vi "DriveModuleOpen.vi"(6 "Magnet Offset (Degrees)":dbl, 7 "ModualNamePrefix":string, 8 "error in":errorcluster, 9 "EncoderCanID":u8, 10 "SpinCanID":u8, 11 "TravelCanID":u8) -> (0 "error out":errorcluster)   [LabVIEW 2023]
uses:
  <vilib>/Rock Robotics/WPI/ThirdParty/REV Robotics/REVLib/Typedef/Spark MAX Idle Mode.ctl
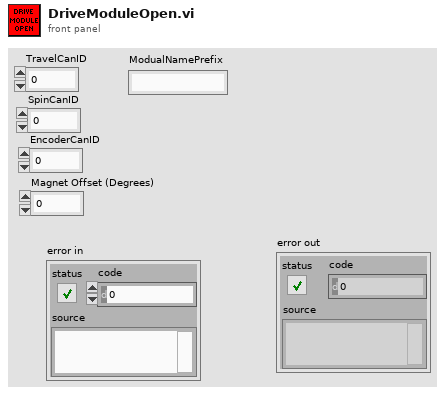
[diagram p1: front panel]
types:
  T1 = typedef "Spark MAX Idle Mode.ctl" = enum16{"Coast", "Brake"}
  T2 = typedef "CTRE_Phoenix_CANcoder_DeviceRef.ctl" = cluster{"DeviceStatus":errorcluster, "Device Number":u8, "Handle":u64, "UsageFrame":u32, "Library Path":path}
  T3 = typedef "WPI_MotorControlDeviceRef.ctl" = cluster{"DeviceStatus":errorcluster, "Type":T4, "PWM":cluster{"PWM Channel":T5, "DeadBand":T6}, "CAN":cluster{"Device Number":u8, "SetOutput VI Ref":variant, "GetOutput VI Ref":variant, "Enable VI Ref":variant, "Disable VI Ref":variant, "Data":variant}, "Invert":bool, "DIO PWM":cluster{"PWM \"Enable\" Channel":T5, "DIOChannel":T7, "PWM Rate":dbl}}
  T4 = typedef "WPI_MotorControlType.ctl" = enum16{"PWM", "CAN", "DIO PWM"}
  T5 = typedef "FPGA_DIOPWMChannel.ctl" = enum8{"PWM 0", "PWM 1", "PWM 2", "PWM 3", "PWM 4", "PWM 5", "PWM 6", "PWM 7", "PWM 8", "PWM 9", "PWM MXP 0", "PWM MXP 1", "PWM MXP 2", "PWM MXP 3", "PWM MXP 4", "PWM MXP 5", "PWM MXP 6", "PWM MXP 7", "PWM MXP 8", "PWM MXP 9", "Invalid"}
  T6 = typedef "WPI_PWMDeadband.ctl" = cluster{"Name":string, "maxPositivePwm":i32, "minPositivePwm":i32, "centerPwm":i32, "maxNegativePwm":i32, "minNegativePwm":i32, "angularRange":u16}
  T7 = typedef "FPGA_DIOChannel.ctl" = enum8{"DIO 0", "DIO 1", "DIO 2", "DIO 3", "DIO 4", "DIO 5", "DIO 6", "DIO 7", "DIO 8", "DIO 9", "DIO MXP 0", "DIO MXP 1", "DIO MXP 2", "DIO MXP 3", "DIO MXP 4", "DIO MXP 5", "DIO MXP 6", "DIO MXP 7", "DIO MXP 8", "DIO MXP 9", "DIO MXP 10", "DIO MXP 11", "DIO MXP 12", "DIO MXP 13", "DIO MXP 14", "DIO MXP 15", "SPI Port CS1", "SPI Port CS2", "SPI Port CS3", "SPI Port MISO", "SPI Port MOSI", "Invalid"}
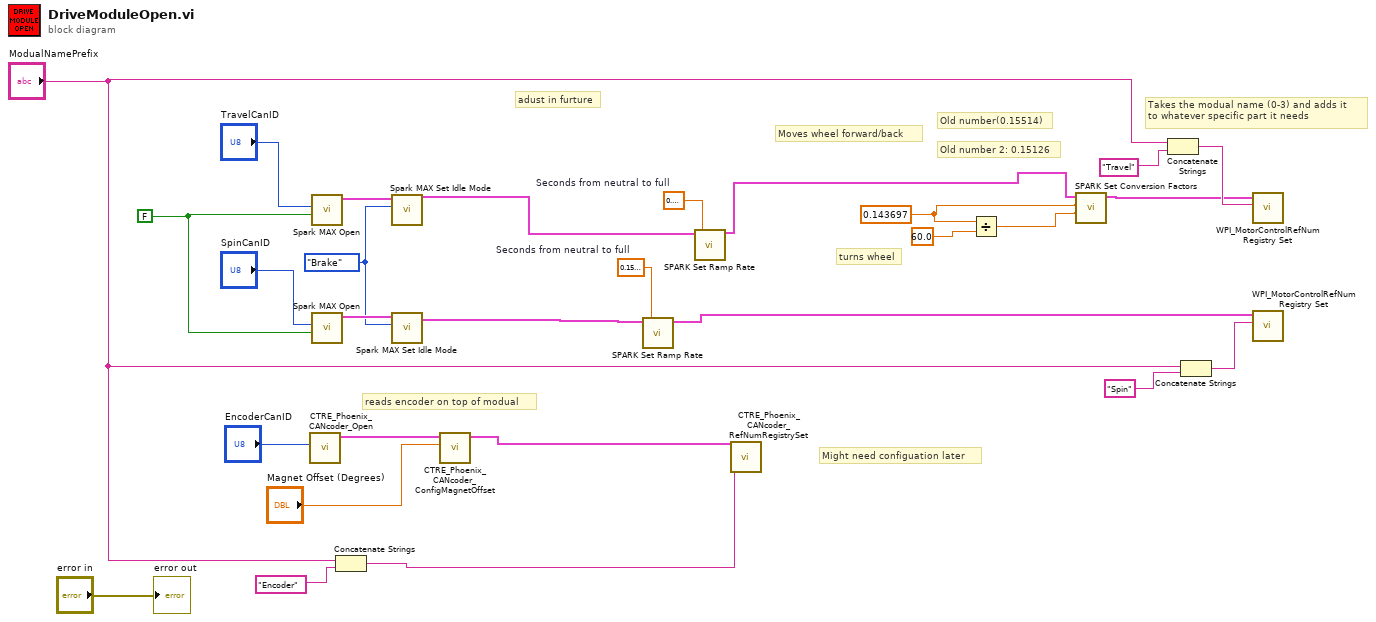
[diagram p0: block diagram]
diagram:
  w5 = sgl 0.15  # Seconds from neutral to full
  w9 = sgl 0.3  # Seconds from neutral to full
  w1 = 0.143697 ("Position Factor (1)")
  w19 = Spark_MAX_Idle_Mode."Brake" ("Idle Mode")
  w28 = FALSE ("Invert")
  # "adust in furture"
  # "Old number 2: 0.15126"
  # "Old number(0.15514)"
  # "reads encoder on top of modual"
  # "turns wheel"
  # "Moves wheel forward/back"
  # "Might need configuation later"
  # "Takes the modual name (0-3) and adds it \nto whatever specific part it needs"
  n1 = call <vilib>:"CTRE_Phoenix_CANcoder_Open.vi"("Device Number"="EncoderCanID") -> ("CTRE_CANcoder_DeviceRef"=w12:T2)  [unwired: 9 in, 1 out]
  n2 = call <vilib>:"Spark MAX Open.vi"("Invert"=w28, "Device Number"="TravelCanID") -> ("MotorControlDeviceRef"=w24:T3)  [unwired: 8 in, 1 out]
  n3 = call <vilib>:"Spark MAX Open.vi"("Invert"=w28, "Device Number"="SpinCanID") -> ("MotorControlDeviceRef"=w25:T3)  [unwired: 8 in, 1 out]
  n4 = Concatenate Strings("ModualNamePrefix", "Encoder" ("refnum name")) -> (w15:string)
  n5 = call <vilib>:"Spark MAX Set Idle Mode.vi"("Idle Mode"=w19, "MotorControlDeviceRef in"=w24) -> ("MotorControlDeviceRef out"=w8:T3)  [unwired: 8 in, 1 out]
  n6 = call <vilib>:"Spark MAX Set Idle Mode.vi"("Idle Mode"=w19, "MotorControlDeviceRef in"=w25) -> ("MotorControlDeviceRef out"=w7:T3)  [unwired: 8 in, 1 out]
  n7 = call <vilib>:"CTRE_Phoenix_CANcoder_ConfigMagnetOffset.vi"("Magnet Offset (Degrees)"="Magnet Offset (Degrees)", "CTRE_CANcoder_DeviceRef"=w12) -> ("CTRE_CANcoder_DeviceRef"=w11:T2)  [unwired: 8 in, 1 out]
  n8 = call <vilib>:"SPARK Set Ramp Rate.vi"("Seconds from neutral to full (0)"=w5, "MotorControlDeviceRef in"=w7) -> ("MotorControlDeviceRef"=w6:T3)  [unwired: 8 in, 1 out]
  n9 = call <vilib>:"SPARK Set Ramp Rate.vi"("Seconds from neutral to full (0)"=w9, "MotorControlDeviceRef in"=w8) -> ("MotorControlDeviceRef"=w4:T3)  [unwired: 8 in, 1 out]
  n10 = call <vilib>:"CTRE_Phoenix_CANcoder_RefNumRegistrySet.vi"("refnum name"=w15, "CTRE_CANcoder_DeviceRef"=w11) -> ()  [unwired: 8 in, 2 out]
  n11 = Divide(x=w1, y=60.0) -> (x/y=w2:dbl)
  n12 = call <vilib>:"SPARK Set Conversion Factors.vi"("Velocity Factor (1)"=w2, "Position Factor (1)"=w1, "MotorControlDeviceRef in"=w4) -> ("MotorControlDeviceRef out"=w3:T3)  [unwired: 7 in, 1 out]
  n13 = Concatenate Strings("ModualNamePrefix", "Travel" ("refnum name")) -> (w22:string)
  n14 = Concatenate Strings("ModualNamePrefix", "Spin" ("refnum name")) -> (w20:string)
  n15 = call <vilib>:"WPI_MotorControlRefNum Registry Set.vi"("refnum name"=w22, "MotorControlDevRef"=w3) -> ()  [unwired: 8 in, 2 out]
  n16 = call <vilib>:"WPI_MotorControlRefNum Registry Set.vi"("refnum name"=w20, "MotorControlDevRef"=w6) -> ()  [unwired: 8 in, 2 out]
  "error out" <- "error in"
